vi "Config File Save.vi"(0 "String in":refnum<vi>, 1 "Channel 5":T1={"Port No."="", "Checkbox"=FALSE, "Parity"=0, "Stop Bit"=0, "Baud Rate"=9600, "Data Bits"=8} {"Stop Bit" items=["1.0", "1.5", "2.0"]; "Parity" items=["None", "Odd", "Even", "Mark", "Space"]}, 2 "Channel 6":T1={"Port No."="", "Checkbox"=FALSE, "Parity"=0, "Stop Bit"=0, "Baud Rate"=9600, "Data Bits"=8} {"Stop Bit" items=["1.0", "1.5", "2.0"]; "Parity" items=["None", "Odd", "Even", "Mark", "Space"]}, 3 "Channel 7":T1={"Port No."="", "Checkbox"=FALSE, "Parity"=0, "Stop Bit"=0, "Baud Rate"=9600, "Data Bits"=8} {"Stop Bit" items=["1.0", "1.5", "2.0"]; "Parity" items=["None", "Odd", "Even", "Mark", "Space"]}, 4 "Channel 8":T1={"Port No."="", "Checkbox"=FALSE, "Parity"=0, "Stop Bit"=0, "Baud Rate"=9600, "Data Bits"=8} {"Stop Bit" items=["1.0", "1.5", "2.0"]; "Parity" items=["None", "Odd", "Even", "Mark", "Space"]}, 5 "Channel 1":T1={"Port No."="", "Checkbox"=FALSE, "Parity"=0, "Stop Bit"=0, "Baud Rate"=9600, "Data Bits"=8} {"Stop Bit" items=["1.0", "1.5", "2.0"]; "Parity" items=["None", "Odd", "Even", "Mark", "Space"]}, 6 "Configuration Folder Path":path=path "D:/BEL_FCS_Project/FCTS_JIG_LV/Configuration Files/Port Configuration", 7 "Channel 4":T1={"Port No."="", "Checkbox"=FALSE, "Parity"=0, "Stop Bit"=0, "Baud Rate"=9600, "Data Bits"=8} {"Stop Bit" items=["1.0", "1.5", "2.0"]; "Parity" items=["None", "Odd", "Even", "Mark", "Space"]}, 9 "Channel 2":T1={"Port No."="", "Checkbox"=FALSE, "Parity"=0, "Stop Bit"=0, "Baud Rate"=9600, "Data Bits"=8} {"Stop Bit" items=["1.0", "1.5", "2.0"]; "Parity" items=["None", "Odd", "Even", "Mark", "Space"]}, 11 "Channel 3":T1={"Port No."="", "Checkbox"=FALSE, "Parity"=0, "Stop Bit"=0, "Baud Rate"=9600, "Data Bits"=8} {"Stop Bit" items=["1.0", "1.5", "2.0"]; "Parity" items=["None", "Odd", "Even", "Mark", "Space"]}, 12 "Save":bool) -> (15 "File Name":string)   [LabVIEW 2020]
uses:
  Port details.ctl
panel:
  in  "error in (no error)":errorcluster
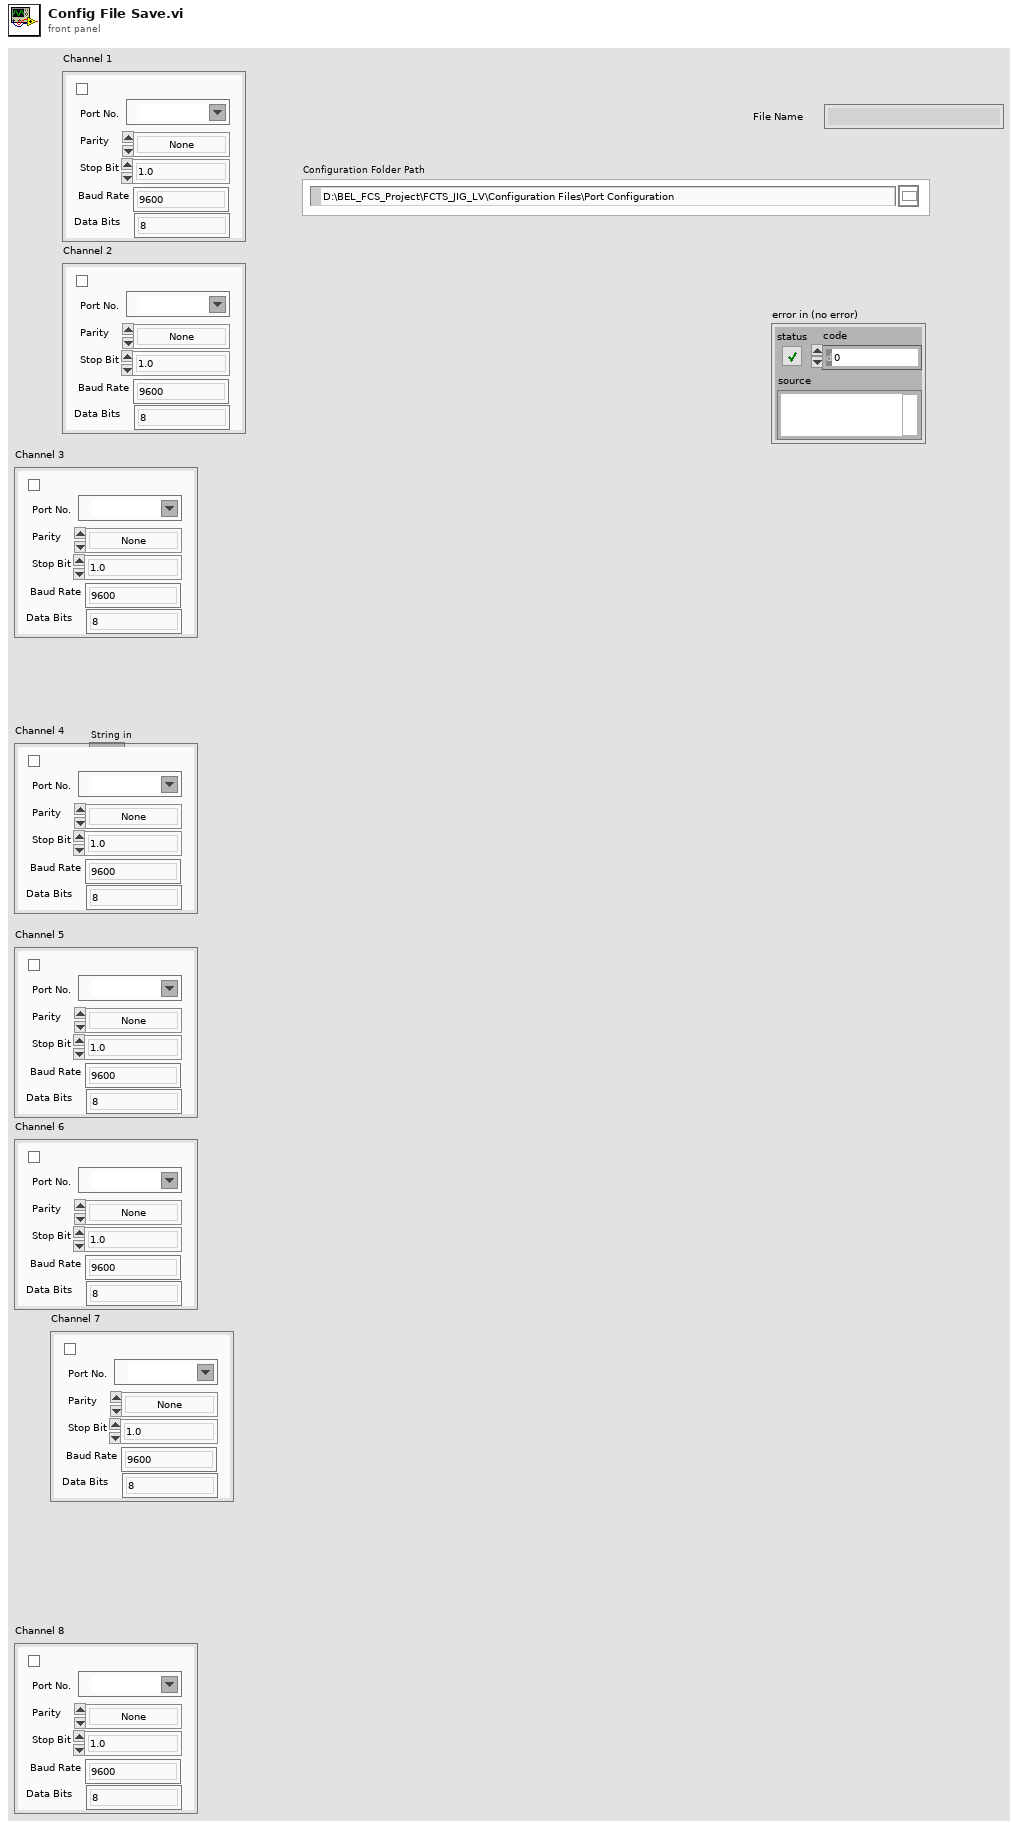
[diagram p1: front panel]
types:
  T1 = typedef "Port details.ctl" = cluster{"Port No.":refnum<visa-resource-name>, "Checkbox":bool, "Parity":u16, "Stop Bit":u16, "Baud Rate":u32, "Data Bits":u8}
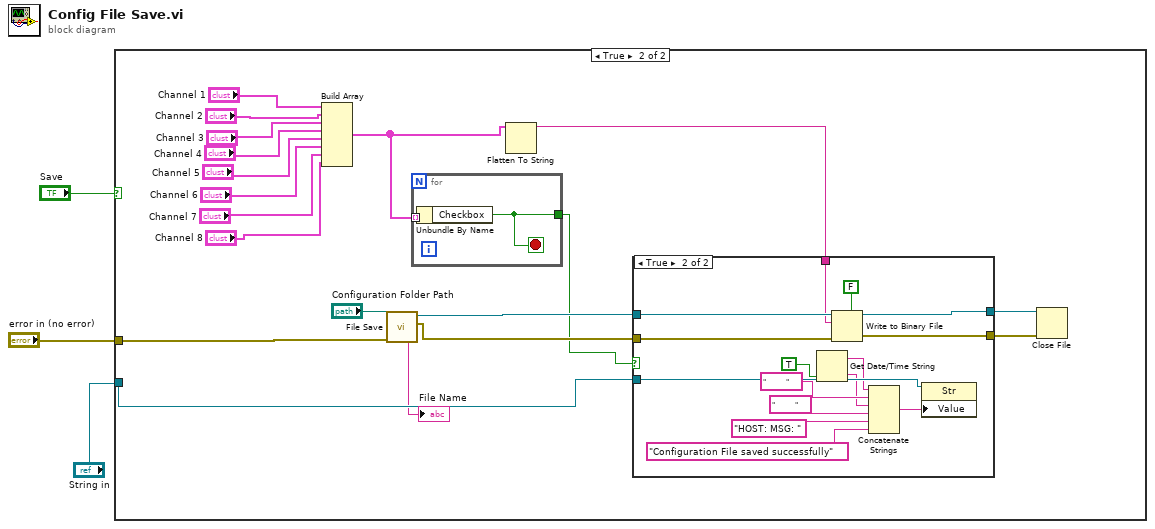
[diagram p0: block diagram]
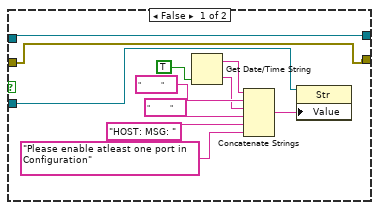
[diagram p3: hidden frame]
diagram:
  n1 = case shown="True" "Save" {
    tunnel: "error in (no error)" -> [_ w19]
    tunnel: "String in" -> [_ w22]
    frame False {
    }
    frame True {
      n2 = Build Array("Channel 1", "Channel 2", "Channel 3", "Channel 4", "Channel 5", "Channel 6", "Channel 7", "Channel 8") -> (w7:T1[])
      n3 = call "File Save.vi"("error in"=w19, "Path"="Configuration Folder Path") -> ("error out"=w20:errorcluster, "refnum out"=w21:refnum<file>, "File Name 2"=→"File Name":string)  [unwired: 6 in, 1 out]
      n4 = for {
        tunnel: w7 -> [w50] mode=indexing
        tunnel: [w49] -> w6
        stop <- w49 stop-if-true
        n5 = Unbundle By Name(w50) -> ("Checkbox"=w49:bool)
      }
      n6 = Flatten To String(anything=w7) -> (data string=w8:string)  [unwired: 3 in, 2 out]
      n7 = case shown="True" w6 {
        tunnel: w22 -> [w24 w48]
        tunnel: [w33 w47] -> w5
        tunnel: w21 -> [w33 w46]
        tunnel: w20 -> [w23 w45]
        tunnel: [w23 w36] -> w4
        tunnel: w8 -> [_ w34]
        frame False {
          n8 = Get Date/Time String(want seconds? (F)=TRUE) -> (date string=w27:string, time string=w26:string)  [unwired: 2 in]
          n9 = Concatenate Strings(w27, "          ", w26, "          ", "HOST: MSG: " ("string"), "Please enable atleast one port in Configuration" ("String")) -> (w25:string)
          n10 = property class="Str"(reference=w24, "Value"=w25) -> ()  [unwired: 1 in, 2 out]
        }
        frame True {
          n11 = Get Date/Time String(want seconds? (F)=TRUE) -> (date string=w39:string, time string=w38:string)  [unwired: 2 in]
          n12 = Write to Binary File(file (use dialog)=w46, data=w34, error in=w45, 5:FALSE ("prepend array or string size? (T)")) -> (refnum out=w47:refnum<file>, error out=w36:errorcluster)  [unwired: 2 in, 1 out]
          n13 = Concatenate Strings(w39, "          ", w38, "          ", "HOST: MSG: " ("string"), "Configuration File saved successfully" ("String")) -> (w37:string)
          n14 = property class="Str"(reference=w48, "Value"=w37) -> ()  [unwired: 1 in, 2 out]
        }
      }
      n15 = Close File(refnum=w5, error in=w4) -> ()  [unwired: 2 out]
    }
  }
